vi "Write Voltage Data to Optimization (Off-Grid).vi"(5 "Network Data Array":T1[](array[typedef]), 7 "Bus by ID":T2[](array[typedef]), 8 "error in":errorcluster, 11 "Off-Grid Optimization in":refnum<class "Off-Grid.lvclass">) -> (0 "error out":errorcluster, 3 "Off-Grid Optimization out":refnum<class "Off-Grid.lvclass">)   [LabVIEW 2018, in "Off-Grid Actor.lvlib" / "Off-Grid.lvclass"]
uses:
  Off-Grid.lvclass
  C:/Users/Administrator/Desktop/LabVIEW EMS/EMS Generic Actor/EMS Generic/EMS Generic.lvclass
  C:/Users/Administrator/Desktop/LabVIEW EMS/Optimization/Generic Optimization Actor/Generic Optimization/Generic Optimization.lvclass
  Generic Optimization Actor/Generic Optimization/Optimization Controls/Bus by ID.ctl
  <vilib>/ORNL/CSEISMIC DDS/CSEISMIC DDS Base/Data Types/Controls/DeviceID.ctl
  Generic Optimization Actor/Generic Optimization/Optimization Controls/Electrical Network Optimization Data.ctl
  EMS Generic Actor/EMS Generic/EMS Generic.lvclass/EMS Generic.ctl
  Generic Optimization Actor/Generic Optimization/Optimization Controls/Bus Voltage.ctl
  <vilib>/ORNL/CSEISMIC DDS/CSEISMIC DDS Base/Data Types/SmartRelay_Measurement.ctl
  <vilib>/ORNL/CSEISMIC DDS/CSEISMIC DDS Base/Data Types/DER_Measurement.ctl
  <vilib>/ORNL/CSEISMIC DDS/CSEISMIC DDS Base/Data Types/Meter_Measurement.ctl
  Global Variables/Global Variables.vi
  <vilib>/ORNL/CSEISMIC DDS/CSEISMIC DDS Base/CSEISMIC DDS.lvclass
  EMS Generic Actor/EMS Generic/EMS Generic.lvclass
  Generic Optimization Actor/Generic Optimization/Generic Optimization.lvclass
  <vilib>/Analysis/NI_AALBase.lvlib
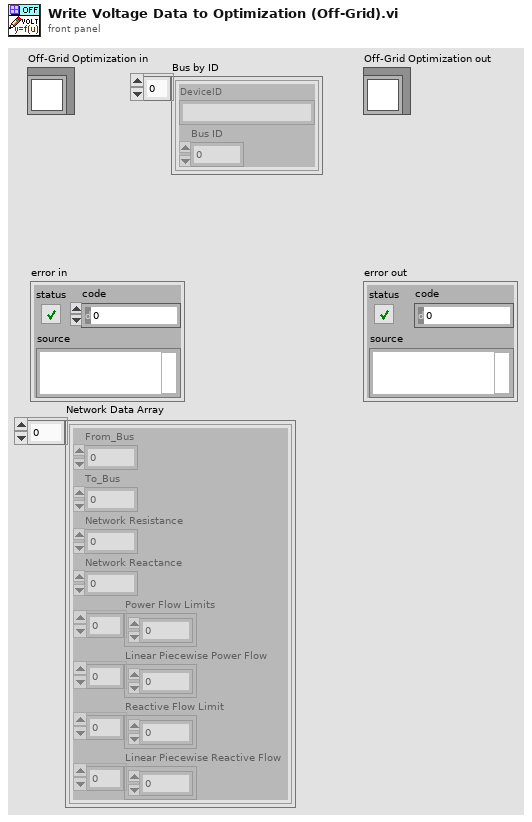
[diagram p1: front panel]
types:
  T1 = typedef "Generic Optimization Actor.lvlib/Generic Optimization.lvclass/Electrical Network Optimization Data.ctl" = cluster{"From_Bus":dbl, "To_Bus":dbl, "Network Resistance":dbl, "Network Reactance":dbl, "Power Flow Limits":dbl[], "Linear Piecewise Power Flow":dbl[], "Reactive Flow Limit":dbl[], "Linear Piecewise Reactive Flow":dbl[]}
  T2 = typedef "Generic Optimization Actor.lvlib/Generic Optimization.lvclass/Bus by ID.ctl" = cluster{"DeviceID":T3, "Bus ID":dbl}
  T3 = typedef "CSEISMIC DDS.lvlib/CSEISMIC DDS.lvclass/DeviceID.ctl" = string
  T4 = typedef "Generic Optimization Actor.lvlib/Generic Optimization.lvclass/Bus Voltage.ctl" = cluster{"Bus":dbl, "Voltage":dbl}
  T5 = typedef "CSEISMIC DDS.lvlib/CSEISMIC DDS.lvclass/Meter_Measurement.ctl" = cluster{"DeviceID":T3, "Voltage":dbl[], "Current":dbl[], "RealPower":dbl[], "ReactivePower":dbl[], "LineConfig":u8[], "Frequency":dbl}
  T6 = typedef "CSEISMIC DDS.lvlib/CSEISMIC DDS.lvclass/SmartRelay_Measurement.ctl" = cluster{"DeviceID":T3, "PrimaryVoltage":dbl[], "SecondaryVoltage":dbl[], "Current":dbl[], "RealPower":dbl[], "ReactivePower":dbl[], "LineConfig":u8[], "Frequency":dbl}
  T7 = typedef "CSEISMIC DDS.lvlib/CSEISMIC DDS.lvclass/DER_Measurement.ctl" = cluster{"DeviceID":T3, "Voltage":dbl[], "Current":dbl[], "RealPower":dbl[], "ReactivePower":dbl[], "LineConfig":u8[], "Frequency":dbl}
  T8 = typedef "EMS Generic Actor.lvlib/EMS Generic.lvclass/Data Type DVRs.ctl" = cluster{"IED_Status":refnum<data-value>, "IED_Status_0":refnum<data-value>, "DER_Measurement":refnum<data-value>, "DER_Info":refnum<data-value>, "DER_Status":refnum<data-value>, "ES_Measurement":refnum<data-value>, "ES_Info":refnum<data-value>, "PV_Info":refnum<data-value>, "SmartRelay_Info":refnum<data-value>, "SmartRelay_Measurement":refnum<data-value>, "Meter_Info":refnum<data-value>, "Meter_Measurement":refnum<data-value>, "HVAC_Status":refnum<data-value>, "HVAC_Measurement":refnum<data-value>, "PriceData_RealTime":refnum<data-value>, "PriceData_Demand":refnum<data-value>, "PriceData_Energy":refnum<data-value>, "ForecastData_Long":refnum<data-value>, "ForecastData_Short":refnum<data-value>, "DER_Control":refnum<data-value>, "DER_SetPointF":refnum<data-value>, "DER_SetPointP":refnum<data-value>, "DER_SetPointQ":refnum<data-value>, "DER_SetPointPF":refnum<data-value>, "DER_SetPointV":refnum<data-value>, "PV_setCurtailment":refnum<data-value>, "PV_setRampRate":refnum<data-value>, "Relay_Control":refnum<data-value>, "Load_Control":refnum<data-value>, "HVAC_Control":refnum<data-value>, "Generator_Info":refnum<data-value>, "ForecastData_Long_Backup":refnum<data-value>, "PriceData_RealTime_Backup":refnum<data-value>}
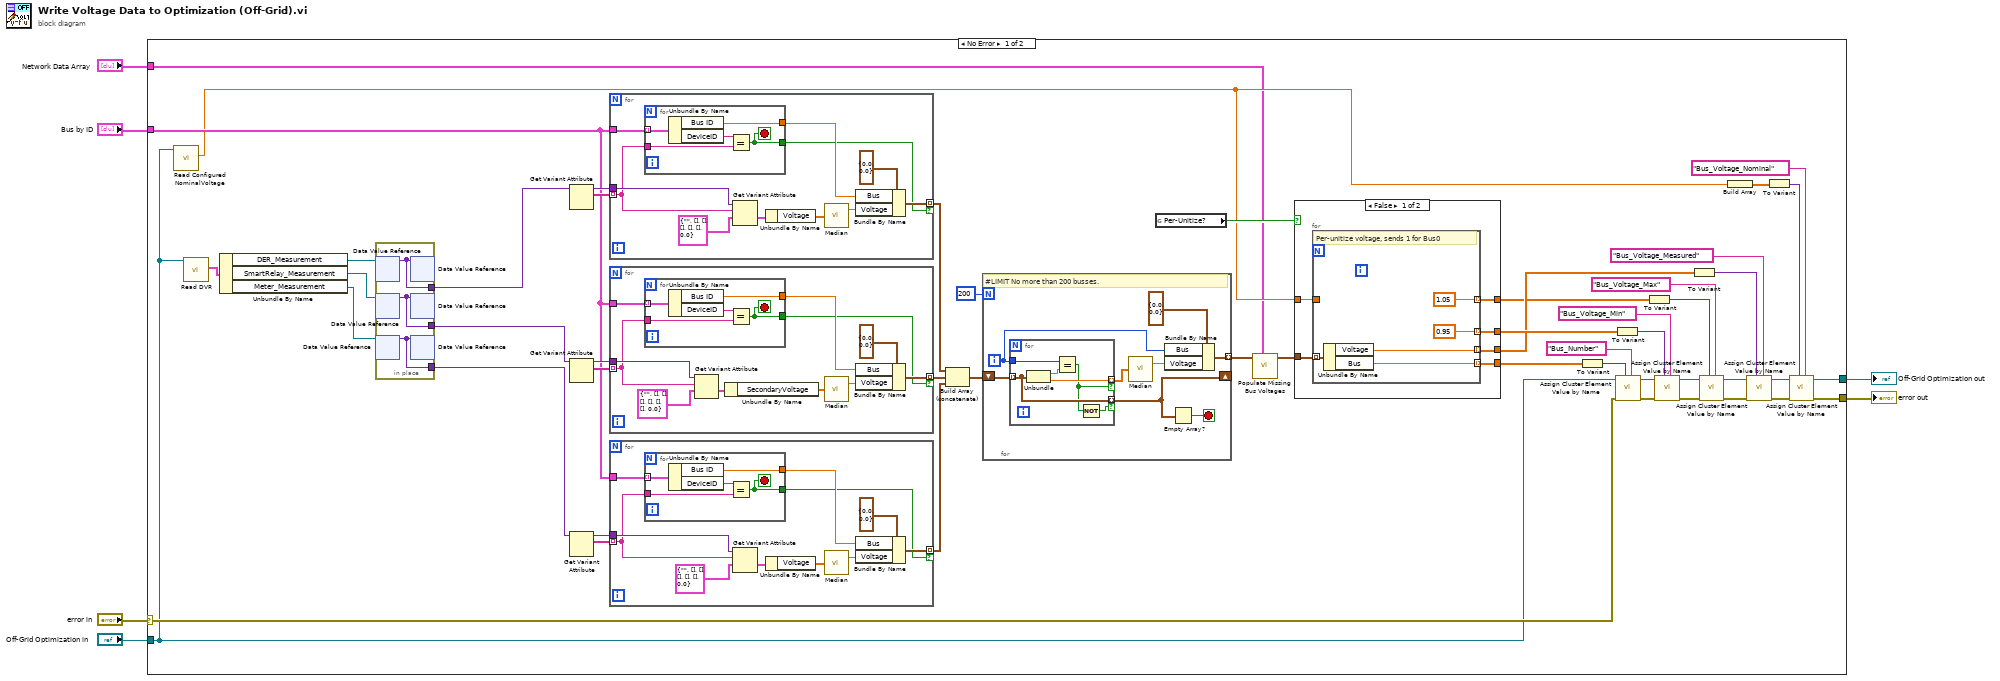
[diagram p0: block diagram]
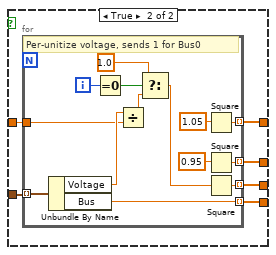
[diagram p2: hidden frame]
diagram:
  n1 = case shown="No Error" "error in" {
    selector: "error in" -> [w43 w155]
    tunnel: [w14 w155] -> w6
    tunnel: "Bus by ID" -> [w25 _]
    tunnel: "Off-Grid Optimization in" -> [w8 w154]
    tunnel: [w7 w154] -> w2
    tunnel: "Network Data Array" -> [w9 _]
    frame No Error {
      n2 = call "Read Configured NominalVoltage.vi"("EMS Generic in"=w8) -> ("NominalVoltage"=w12:dbl)  [unwired: 8 in, 2 out]
      n3 = call "Read DVR.vi"("EMS Generic in"=w8) -> ("DVR"=w39:T8)  [unwired: 9 in, 1 out]
      n4 = Unbundle By Name(w39) -> ("DER_Measurement"=w38:refnum<data-value>, "SmartRelay_Measurement"=w37:refnum<data-value>, "Meter_Measurement"=w24:refnum<data-value>)
      n5 = in-place {
        in-place-border: [w153] -> w23
        in-place-border: [w152] -> w22
        in-place-border: [w151] -> w21
        n6 = in-place-dvr #1(w38) -> (w153:variant)  [unwired: 1 out]
        n7 = in-place-dvr #2(w37) -> (w152:variant)  [unwired: 1 out]
        n8 = in-place-dvr #3(w24) -> (w151:variant)  [unwired: 1 out]
        n9 = in-place-dvr #1(w153) -> ()  [unwired: 2 out]
        n10 = in-place-dvr #2(w152) -> ()  [unwired: 2 out]
        n11 = in-place-dvr #3(w151) -> ()  [unwired: 2 out]
      }
      n12 = Get Variant Attribute(Variant=w23) -> (duplicate Variant=w35:variant, names=w36:string[])  [unwired: 3 in, 2 out]
      n13 = Get Variant Attribute(Variant=w22) -> (duplicate Variant=w34:variant, names=w33:string[])  [unwired: 3 in, 2 out]
      n14 = Get Variant Attribute(Variant=w21) -> (duplicate Variant=w31:variant, names=w32:string[])  [unwired: 3 in, 2 out]
      n15 = for {
        tunnel: w36 -> [w143] mode=indexing
        tunnel: w35 -> [w145]
        tunnel: w25 -> [w144]
        tunnel: [w141] -> w30 mode=indexing if=w135
        n16 = for {
          tunnel: w144 -> [w150] mode=indexing
          tunnel: w143 -> [w149]
          tunnel: [w147] -> w137
          tunnel: [w146] -> w135
          stop <- w146 stop-if-true
          n17 = Unbundle By Name(w150) -> ("Bus ID"=w147:dbl, "DeviceID"=w148:T3)
          n18 = Equal?(x=w148, y=w149) -> (x = y?=w146:bool)
        }
        n19 = Get Variant Attribute(Variant=w145, name=w143, default value (empty Variant)=T7 {"DeviceID"="", "Voltage"=[], "Current"=[], "RealPower"=[], "ReactivePower"=[], "LineConfig"=[], "Frequency"=0.0} ("DER_Measurement")) -> (value=w142:T7)  [unwired: 1 in, 3 out]
        n20 = Unbundle By Name(w142) -> ("Voltage"=w139:dbl[])
        n21 = call <vilib>:"Median.vi"("X"=w139) -> ("median"=w138:dbl)  [unwired: 1 out]
        n22 = Bundle By Name(cluster=T4 {"Bus"=0.0, "Voltage"=0.0} ("Bus Voltage"), "Bus"=w137, "Voltage"=w138) -> (w141:T4)
      }
      n23 = for {
        tunnel: w33 -> [w127] mode=indexing
        tunnel: w34 -> [w129]
        tunnel: w25 -> [w128]
        tunnel: [w125] -> w29 mode=indexing if=w120
        n24 = for {
          tunnel: w128 -> [w134] mode=indexing
          tunnel: w127 -> [w133]
          tunnel: [w131] -> w122
          tunnel: [w130] -> w120
          stop <- w130 stop-if-true
          n25 = Unbundle By Name(w134) -> ("Bus ID"=w131:dbl, "DeviceID"=w132:T3)
          n26 = Equal?(x=w132, y=w133) -> (x = y?=w130:bool)
        }
        n27 = Get Variant Attribute(Variant=w129, name=w127, default value (empty Variant)=T6 {"DeviceID"="", "PrimaryVoltage"=[], "SecondaryVoltage"=[], "Current"=[], "RealPower"=[], "ReactivePower"=[], "LineConfig"=[], "Frequency"=0.0} ("SmartRelay_Measurement")) -> (value=w126:T6)  [unwired: 1 in, 3 out]
        n28 = Unbundle By Name(w126) -> ("SecondaryVoltage"=w124:dbl[])
        n29 = call <vilib>:"Median.vi"("X"=w124) -> ("median"=w123:dbl)  [unwired: 1 out]
        n30 = Bundle By Name(cluster=T4 {"Bus"=0.0, "Voltage"=0.0} ("Bus Voltage"), "Bus"=w122, "Voltage"=w123) -> (w125:T4)
      }
      n31 = for {
        tunnel: w32 -> [w111] mode=indexing
        tunnel: w31 -> [w113]
        tunnel: w25 -> [w112]
        tunnel: [w109] -> w28 mode=indexing if=w104
        n32 = for {
          tunnel: w112 -> [w118] mode=indexing
          tunnel: w111 -> [w117]
          tunnel: [w115] -> w106
          tunnel: [w114] -> w104
          stop <- w114 stop-if-true
          n33 = Unbundle By Name(w118) -> ("Bus ID"=w115:dbl, "DeviceID"=w116:T3)
          n34 = Equal?(x=w116, y=w117) -> (x = y?=w114:bool)
        }
        n35 = Get Variant Attribute(Variant=w113, name=w111, default value (empty Variant)=T5 {"DeviceID"="", "Voltage"=[], "Current"=[], "RealPower"=[], "ReactivePower"=[], "LineConfig"=[], "Frequency"=0.0} ("Meter_Measurement")) -> (value=w110:T5)  [unwired: 1 in, 3 out]
        n36 = Unbundle By Name(w110) -> ("Voltage"=w108:dbl[])
        n37 = call <vilib>:"Median.vi"("X"=w108) -> ("median"=w107:dbl)  [unwired: 1 out]
        n38 = Bundle By Name(cluster=T4 {"Bus"=0.0, "Voltage"=0.0} ("Bus Voltage"), "Bus"=w106, "Voltage"=w107) -> (w109:T4)
      }
      n39 = Build Array (concatenate)(w30, w29, w28) -> (w27:T4[])
      n40 = for {
        N: 200 -> [_]
        shift-right: [w95] -> _
        shift-left: w27 -> [w96]
        tunnel: [w89] -> w11 mode=indexing
        i -> [w91]
        stop <- w94 stop-if-true
        # "#LIMIT No more than 200 busses."
        n41 = for {
          tunnel: w96 -> [w99] mode=indexing
          tunnel: w91 -> [w102]
          tunnel: [w100] -> w93 mode=indexing if=w98
          tunnel: [w99] -> w95 mode=indexing if=w97
          n42 = Unbundle(w99) -> ("Bus"=w101:dbl, "Voltage"=w100:dbl)
          n43 = Equal?(x=w102, y=w101) -> (x = y?=w98:bool)
          n44 = Not(x=w98) -> (.not. x?=w97:bool)
        }
        n45 = call <vilib>:"Median.vi"("X"=w93) -> ("median"=w90:dbl)  [unwired: 1 out]
        n46 = Bundle By Name(cluster=T4 {"Bus"=0.0, "Voltage"=0.0} ("Bus Voltage"), "Bus"=w91, "Voltage"=w90) -> (w89:T4)
        n47 = Empty Array?(array=w95) -> (empty?=w94:bool)
      }
      n48 = global read "Global Variables.vi" "Per-Unitize?"() -> (w19:bool)
      n49 = call "Populate Missing Bus Voltages.vi"("Network Data Array"=w9, "Bus Voltage Array in"=w11) -> ("Bus Voltage Array out"=w10:T4[])  [unwired: 8 in, 1 out]
      n50 = case shown="False" w19 {
        tunnel: [w63 w69] -> w42
        tunnel: [w62 w71] -> w41
        tunnel: [w60 w70] -> w40
        tunnel: w10 -> [w59 w74]
        tunnel: w12 -> [w58 w73]
        tunnel: [w61 w72] -> w20
        frame False {
          n51 = for {
            tunnel: w59 -> [w68] mode=indexing
            tunnel: [w66] -> w60 mode=indexing
            tunnel: w58 -> [_]
            tunnel: [1.05 ("x")] -> w61 mode=indexing
            tunnel: [0.95 ("x")] -> w62 mode=indexing
            tunnel: [w67] -> w63 mode=indexing
            # "Per-unitize voltage, sends 1 for Bus0"
            n52 = Unbundle By Name(w68) -> ("Voltage"=w66:dbl, "Bus"=w67:dbl)
          }
        }
        frame True {
          n53 = for {
            tunnel: w74 -> [w88] mode=indexing
            tunnel: [w87] -> w70 mode=indexing
            tunnel: w73 -> [w76]
            tunnel: [w86] -> w72 mode=indexing
            tunnel: [w85] -> w71 mode=indexing
            tunnel: [w84] -> w69 mode=indexing
            i -> [w78]
            # "Per-unitize voltage, sends 1 for Bus0"
            n54 = Unbundle By Name(w88) -> ("Voltage"=w77:dbl, "Bus"=w84:dbl)
            n55 = Equal To 0?(x=w78) -> (x = 0?=w83:bool)
            n56 = Divide(x=w77, y=w76) -> (x/y=w75:dbl)
            n57 = Select(t=1.0, s=w83, f=w75) -> (s? t:f=w82:dbl)
            n58 = Square(x=1.05) -> (x^2=w86:dbl)
            n59 = Square(x=0.95) -> (x^2=w85:dbl)
            n60 = Square(x=w82) -> (x^2=w87:dbl)
          }
        }
      }
      n61 = To Variant(anything=w42) -> (Variant=w44:variant)
      n62 = To Variant(anything=w41) -> (Variant=w46:variant)
      n63 = call "Assign Cluster Element Value by Name.vi"("Element Name"="Bus_Number" ("Keyword Name"), "Value"=w44, "error in"=w43, "Generic Optimization"=w8) -> ("error out"=w55:errorcluster, "Generic Optimization out"=w54:refnum<class "Off-Grid.lvclass">)  [unwired: 6 in]
      n64 = To Variant(anything=w20) -> (Variant=w48:variant)
      n65 = call "Assign Cluster Element Value by Name.vi"("Element Name"="Bus_Voltage_Min" ("Keyword Name"), "Value"=w46, "error in"=w55, "Generic Optimization"=w54) -> ("error out"=w56:errorcluster, "Generic Optimization out"=w53:refnum<class "Off-Grid.lvclass">)  [unwired: 6 in]
      n66 = To Variant(anything=w40) -> (Variant=w50:variant)
      n67 = call "Assign Cluster Element Value by Name.vi"("Element Name"="Bus_Voltage_Max" ("Keyword Name"), "Value"=w48, "error in"=w56, "Generic Optimization"=w53) -> ("error out"=w57:errorcluster, "Generic Optimization out"=w52:refnum<class "Off-Grid.lvclass">)  [unwired: 6 in]
      n68 = Build Array(w12) -> (w18:dbl[])
      n69 = call "Assign Cluster Element Value by Name.vi"("Element Name"="Bus_Voltage_Measured" ("Keyword Name"), "Value"=w50, "error in"=w57, "Generic Optimization"=w52) -> ("error out"=w15:errorcluster, "Generic Optimization out"=w13:refnum<class "Off-Grid.lvclass">)  [unwired: 6 in]
      n70 = To Variant(anything=w18) -> (Variant=w16:variant)
      n71 = call "Assign Cluster Element Value by Name.vi"("Element Name"="Bus_Voltage_Nominal" ("Keyword Name"), "Value"=w16, "error in"=w15, "Generic Optimization"=w13) -> ("error out"=w14:errorcluster, "Generic Optimization out"=w7:refnum<class "Off-Grid.lvclass">)  [unwired: 6 in]
    }
    frame Error {
    }
  }
  "error out" <- w6
  "Off-Grid Optimization out" <- w2
